vi "Soft_Robot Model_2States.vi"() -> ()   [LabVIEW 2015]
uses:
  <vilib>/addons/Control Design/_Model Construction/Model Typedefs.llb/CD State Space Model (MIMO).ctl
  <vilib>/addons/Control Design/_Model Construction/Model Typedefs.llb/CD General Elements.ctl
  <vilib>/Platform/TimedLoop/XDataNode/timing_clust.ctl
  <vilib>/Platform/TimedLoop/XDataNode/nitl_modes.ctl
  <vilib>/Platform/TimedLoop/XDataNode/wakeup.ctl
  <vilib>/FPGAPlugInAG/myRIO-1900/niLvFpga_Open_myRIO-1900.vi
  <vilib>/rvi/interface/common/dynamic/niFpgaDynamicAddResources.vi
  <vilib>/Utility/error.llb/Error Cluster From Error Code.vi
  <vilib>/rvi/errors/niLvFpgaAdjustHostInterfaceError.vi
  <vilib>/FPGAPlugInAG/Dynamic/niLvFpga_Close_Dynamic.vi
  <vilib>/Analysis/7linalg.llb/Create Special Real Matrix.vi
  <vilib>/addons/Control Design/_Model Construction/Model Creation.llb/Model Creation SubVI/cd_Create State Space Model.vi
  <vilib>/addons/Control Design/_State Feedback Control/State Feedback Control.llb/State Feedback Control SubVis/cd_Linear Quadratic Regulator.vi
  <vilib>/addons/Control Design/_Stochastic Systems/Stochastic Systems.llb/CD Construct Noise Model (Numeric).vi
  <vilib>/Simulation/Estimation/Implementation/NILVSim Discrete Kalman Filter.llb/SIM Disc KF Pred and Corr with Pred Gain with Checking Direct LV.vi
  <vilib>/rvi/interface/nirviOpenFPGA/nirviOpenFPGA.xnode
  FPGA Bitfiles/ACC20115_FPGATarget_CurrentControlle_Dt5vFgOzYtY.lvbitx
  Current Controller.vi
  <vilib>/rvi/interface/nirviReadWriteControl/nirviReadWriteControl.xnode
  <vilib>/rvi/interface/nirviCloseFPGA/nirviCloseFPGA.xnode
  <vilib>/Platform/TimedLoop/XDataNode/XDataNode.xnode
  <vilib>/Simulation/Implementation/XNodeFramework/SimXNode/SimX.xnode
  NiFpgaLv.dll
  <vilib>/rvi/interface/Simulation/niFpgaSimulationCallBeginRW.vi
  <vilib>/addons/Control Design/_State Feedback Control/NI_CD_State Feedback Control.lvlib
  <vilib>/addons/Control Design/_Stochastic Systems/NI_CD_Stochastic Systems.lvlib
  <vilib>/Platform/TimedLoop/XDataNode/XDNodeRunTimeDep.lvlib
  <vilib>/Analysis/NI_AALPro.lvlib
  <vilib>/addons/Control Design/_Model Construction/NI_LinSys_Model Creation.lvlib
  <vilib>/addons/Control Design/_Model Construction/NI_LinSys_Model Typedefs.lvlib
panel:
  in  "Tab Control":enum32{"Outputs/Control", "Model Info"}(tab)
  out "DAC Inlet Valve 2":i32(graph)
  out "Fusion Data":dbl(graph)
  out "KF estimate":dbl[](graph)
  in  "SP1:":dbl(slide)=40.87020302841148 min=0.0 max=0.0 scale=0.0..720.0
  in  "Stop":bool
  out "Status?":bool
  in  "Current (mA)":i32
  out "State-Space Model":T1 {"Transport Delay" format="%.2f"; "D" format="%#.2g"; "C" format="%#.2g"; "B" format="%#.2g"; "A" format="%#.2g"; "properties"."Sampling Time" format="%#.6p"; "properties"."Output Delays" format="%.4f"; "properties"."Input Delays" format="%.4f"}
  in  "LQR State Weight Matrix (Q)":dbl[](array[slide])=[1.133823501217849, 15.19911082952933] scale=0.001..1000.0
  in  "LQR Output weighting matrix (R)":dbl[](array[slide])=[0.061359072734131735] scale=0.0001..10.0
  in  "A":dbl[][](array[numeric]) format="%#.5g"
  in  "B":dbl[][](array[numeric]) format="%#.5g"
  in  "C":dbl[][](array[numeric]) format="%#.5g"
  in  "D":dbl[][](array[numeric]) format="%#.5g"
  in  "KF Q":dbl[][](array[numeric]) format="%#.2g"
  in  "KF R":dbl[][](array[numeric]) format="%#.2g"
  in  "KF P(0|-1)":dbl[][](array[numeric])=[[1.0]]
  in  "Stoch. K":dbl[][](array[numeric]) format="%#.2g"
  out "error IO":errorcluster
  in  "xhat(0|-1)":dbl[](array[numeric])=[1.0]
  out "error out":errorcluster
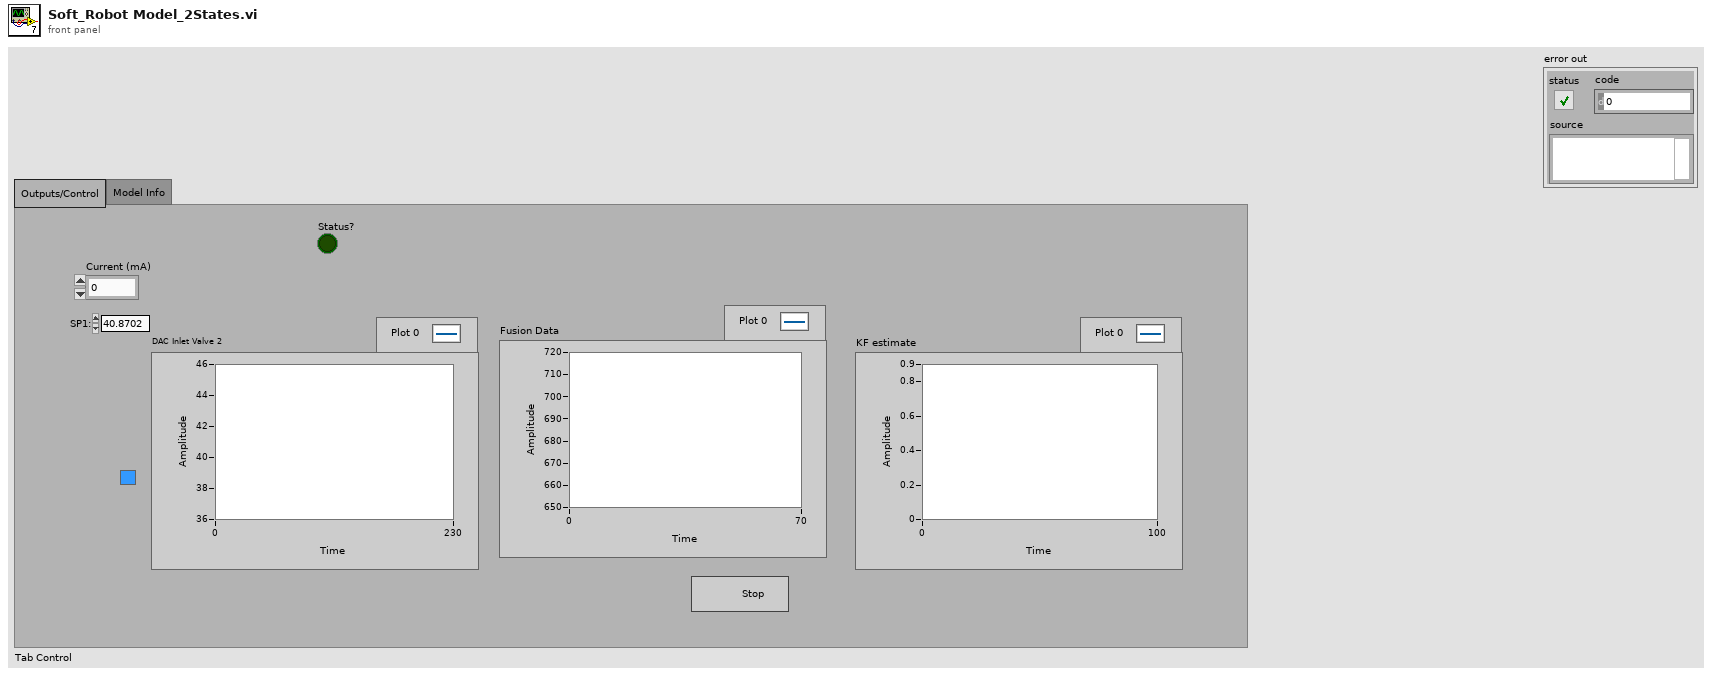
[diagram p1: front panel]
types:
  T1 = typedef "NI_LinSys_Model Typedefs.lvlib/CD State Space Model (MIMO).ctl" = cluster{"properties":T2, "A":dbl[][], "B":dbl[][], "C":dbl[][], "D":dbl[][], "StateNames":string[], "Transport Delay":dbl[][]}
  T2 = typedef "NI_LinSys_Model Typedefs.lvlib/CD General Elements.ctl" = cluster{"Model name":string, "Input names":string[], "Output names":string[], "Input Delays":dbl[], "Output Delays":dbl[], "Sampling Time":dbl, "Notes":string}
  T3 = typedef "XDNodeRunTimeDep.lvlib/timing_clust.ctl" = cluster{"Expected End [f-1]":u64, "Actual End [f-1]":u64, "Finished Late? [f-1]":bool, "Expected End [i-1]":u64, "Actual End [i-1]":u64, "Finished Late? [i-1]":bool, "Expected Start [i]":u64, "Actual Start [i]":u64, "Expected Start [f]":u64, "Actual Start [f]":u64, "Source Name":string, "Structure Name":string, "Period":i64, "Deadline":i64, "Offset":i64, "Start":i64, "Priority":i32, "Timeout":i32, "Mode":T4, "Wakeup Reason":T5, "Error":errorcluster, "Source Type":string, "Secondary Source Type":string, "Global End Time":u64, "Global Start Time":u64, "Frame Duration":u64, "Iteration Duration":u64, "Assigned CPU":i32, "I/O Scan Engine Mode":u32}
  T4 = typedef "XDNodeRunTimeDep.lvlib/nitl_modes.ctl" = enum32{"No Change", "Process missed periods, maintain original phase", "Discard missed periods, maintain original phase", "Process missed periods, ignore original phase", "Discard missed periods, ignore original phase"}
  T5 = typedef "XDNodeRunTimeDep.lvlib/wakeup.ctl" = enum32{"Normal", "Aborted", "Asynchronous wakeup", "Timing source error", "Timed loop error", "Timeout"}
  T6 = enum16{"state weighting", "output weighting, Dim Q = Ny", "output weighting, Dim Q = Nx"}
  T7 = enum32{"Identity", "Diagonal", "Toepliz", "Vandermonde", "Companion"}
  T8 = typedef "NI_Matrix.lvlib/RealMatrix.ctl" = dbl[][]
  T9 = typedef "NI_CD_Stochastic Systems.lvlib/cd_Stochastic State-Space Model.ctl" = cluster{"Sampling Time (s)":dbl, "G":dbl[][], "B":dbl[][], "A":dbl[][], "C":dbl[][], "D":dbl[][], "H":dbl[][]}
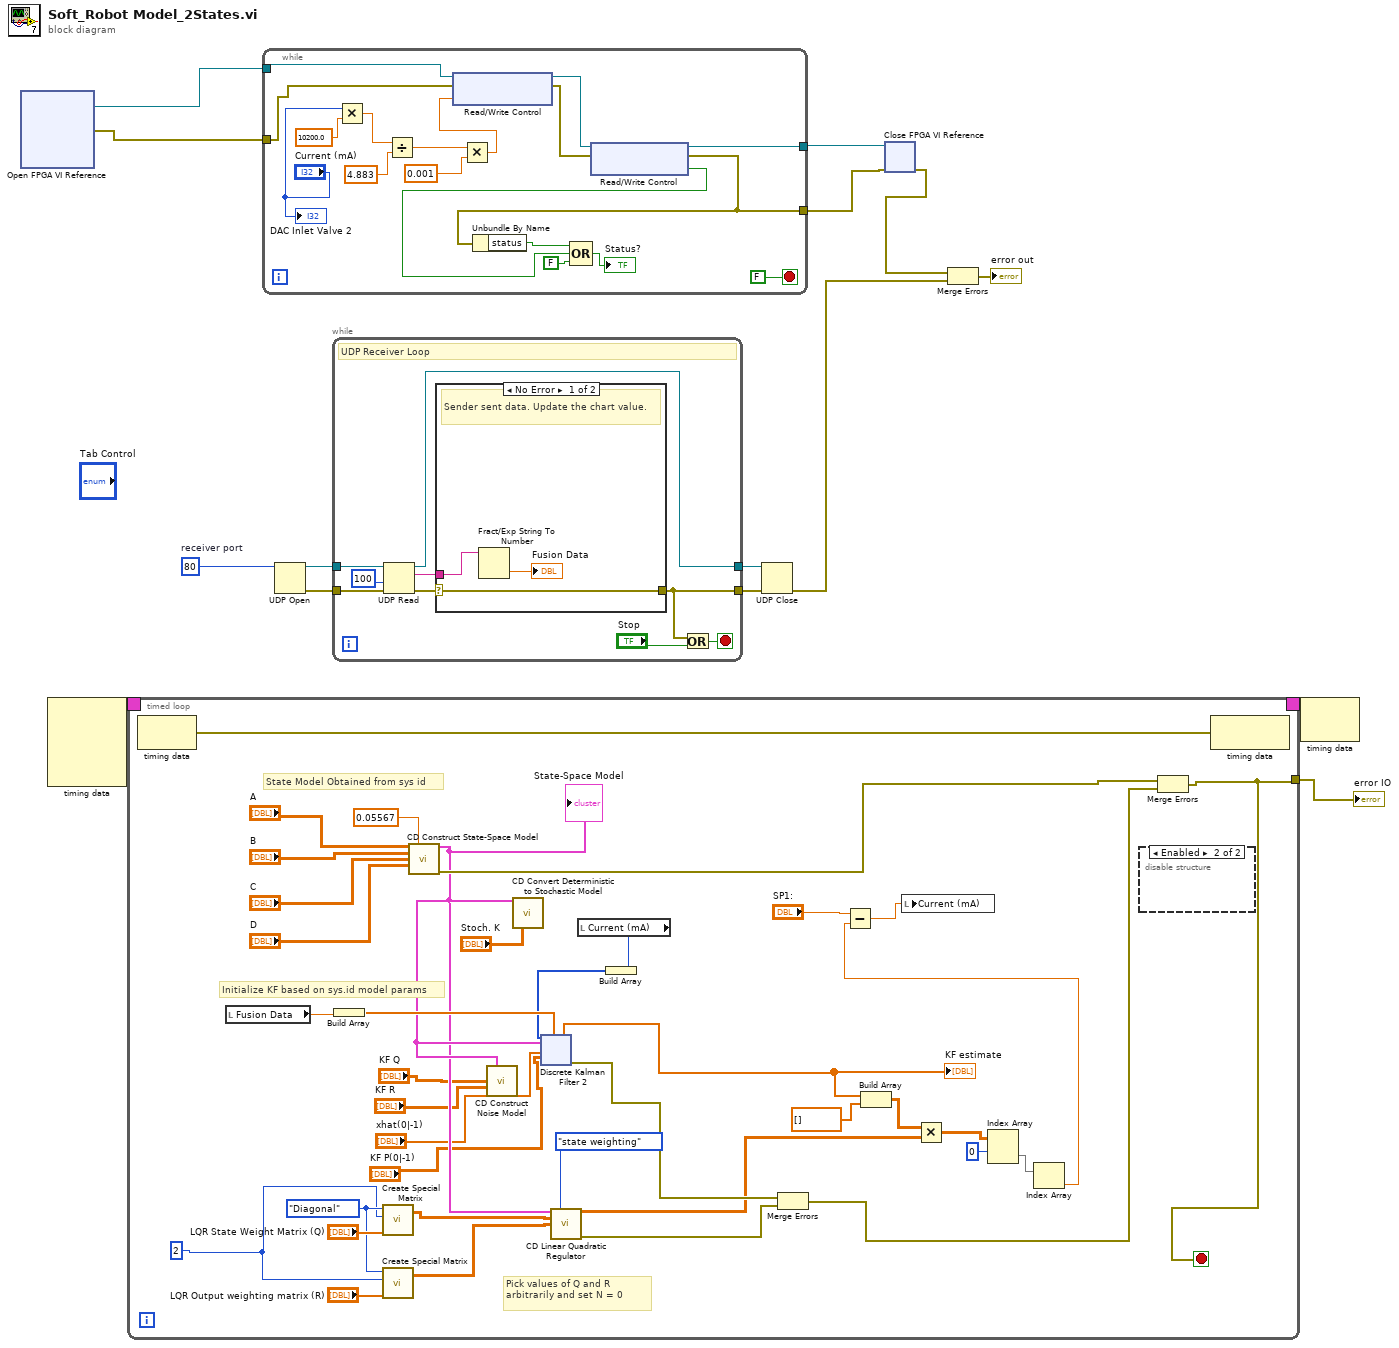
[diagram p0: block diagram]
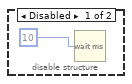
[diagram p2: hidden frame]
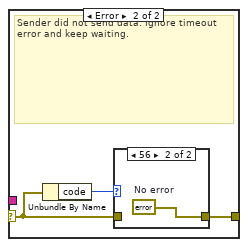
[diagram p3: hidden frame]
diagram:
  w11 = u16 80  # receiver port
  n1 = xnode "Open FPGA VI Reference"() -> ("FPGA VI Reference Out"=w3:refnum<k20>, "error out"=w4:errorcluster)  [unwired: 2 in]
  n2 = node-c288() -> (w2:T3)  [unwired: 4 in]
  n3 = timed-loop {
    tunnel: [w26] -> w5
    timing: w2 -> [_]
    timing-out: [_] -> w1
    stop <- w26 stop-if-true
    w27 = 2
    w34 = T7."Diagonal" ("matrix type")
    # "Pick values of Q and R\narbitrarily and set N = 0"
    # "State Model Obtained from sys id"
    # "Initialize KF based on sys.id model params"
    n4 = node-c288() -> (w25:errorcluster)  [unwired: 1 in]
    n5 = local read "Fusion Data"() -> (w45:dbl)
    n6 = Build Array ("Build Array 6")(w45) -> (w41:dbl[])
    n7 = call-poly <vilib>:"Create Special Matrix.vi"("matrix type"=w34, "matrix size"=w27, "Input Vector1"="LQR State Weight Matrix (Q)") -> ("Special Matrix"=w31:T8)  [unwired: 2 in, 1 out]
    n8 = call-poly <vilib>:"Create Special Matrix.vi"("matrix type"=w34, "matrix size"=w27, "Input Vector1"="LQR Output weighting matrix (R)") -> ("Special Matrix"=w30:T8)  [unwired: 2 in, 1 out]
    n9 = call-poly <vilib>:"CD Construct State-Space Model.vi"("A"="A", "Sampling Time (s)"=0.05567, "B"="B", "C"="C", "D"="D") -> ("State-Space Model"=w32:T1, "error out"=w42:errorcluster)  [unwired: 9 in]
    "State-Space Model" <- w32
    n10 = call <vilib>:"CD Convert Deterministic to Stochastic Model.vi"("Deterministic State-Space Model"=w32, "G"="Stoch. K") -> ("Stochastic State-Space Model"=w38:T9)  [unwired: 12 in, 1 out]
    n11 = call-poly <vilib>:"CD Construct Noise Model.vi"("Stochastic State-Space Model"=w38, "Q"="KF Q", "R"="KF R") -> ()  [unwired: 11 in, 2 out]
    n12 = call-poly <vilib>:"CD Linear Quadratic Regulator.vi"("State-Space Model"=w32, "Weighting Type"=T6."state weighting", "Q"=w31, "R"=w30) -> ("Optimal Gain (K)"=w29:dbl[][], "error out"=w28:errorcluster)  [unwired: 8 in, 2 out]
    n13 = local read "Current (mA)"() -> (w43:i32)
    n14 = Build Array ("Build Array 5")(w43) -> (w37:i32[])
    n15 = xnode ("Discrete Kalman Filter 2")("input u(k)"=w37, "Stochastic State-Space Model"=w38, "Initial State Estimate xhat(0|-1)"="xhat(0|-1)", "Initial Estimation Error Covariance P(0|-1)"="KF P(0|-1)", "Output y(k)"=w41) -> ("Estimated Output yhat(k)"=w40:dbl[], "error out"=w39:errorcluster)  [unwired: 3 in, 6 out]
    "KF estimate" <- w40
    n16 = Merge Errors(w39, w28) -> (w48:errorcluster)
    n17 = Build Array ("Build Array 9")(w40, dbl[] [] ("element")) -> (w50:dbl[][])
    n18 = Multiply(x=w50, y=w29) -> (x*y=w52:dbl[][])
    n19 = Index Array(array=w52, index (row)=0) -> (element=w54:dbl[])  [unwired: 1 in]
    n20 = Index Array ("Index Array 2")(array=w54) -> (element=w46:dbl)  [unwired: 1 in]
    n21 = Subtract(x="SP1:", y=w46) -> (x-y=w44:dbl)
    n22 = local write "Current (mA)"(w44) -> ()
    n23 = disable-structure shown="Enabled" {
      frame Disabled {
        n24 = Wait (ms)(milliseconds to wait=u32 10 ("millisecond timer value")) -> ()  [unwired: 1 out]
      }
      frame Enabled {
      }
    }
    n25 = Merge Errors(w42, w48) -> (w26:errorcluster)
    n26 = node-c288(w25) -> ()  [unwired: 1 out]
  }
  "error IO" <- w5
  n27 = while {
    tunnel: w3 -> [w93]
    tunnel: w4 -> [w77]
    tunnel: [w87] -> w9
    tunnel: [w85] -> w10
    stop <- FALSE stop-if-true
    n28 = Multiply(x="Current (mA)", y=10200.0) -> (x*y=w80:dbl)
    n29 = Divide(x=w80, y=4.883) -> (x/y=w83:dbl)
    n30 = Multiply(x=w83, y=0.001) -> (x*y=w79:dbl)
    n31 = xnode "Read/Write Control"("FPGA VI Reference In"=w93, "error in"=w77, "DAC Inlet Valve"=w79) -> ("FPGA VI Reference Out"=w92:refnum<k20>, "error out"=w91:errorcluster)
    n32 = xnode "Read/Write Control"("FPGA VI Reference In"=w92, "error in"=w91) -> ("FPGA VI Reference Out"=w85:refnum<k20>, "error out"=w87:errorcluster, "Inlet Overflow?"=w86:bool)
    n33 = Unbundle By Name(w87) -> ("status"=w89:bool)
    n34 = Compound Arithmetic op=OR(w89, w86, FALSE ("value")) -> (→"Status?":bool)
    "DAC Inlet Valve 2" <- "Current (mA)"
  }
  n35 = UDP Open(11:w11) -> (port=w12:refnum<k16>, 0:w13:errorcluster)  [unwired: 4 in, 1 out]
  n36 = while {
    tunnel: w12 -> [w103]
    tunnel: [w95] -> w15
    tunnel: w13 -> [w100]
    tunnel: [w96] -> w14
    stop <- w101 stop-if-true
    # "UDP Receiver Loop"
    n37 = UDP Read(connection ID=w103, timeout ms (25000)=100, 8:w100) -> (data out=w98:string, error out=w97:errorcluster, 3:w95:refnum<k16>)  [unwired: 3 out]
    n38 = case shown="No Error" w97 {
      selector: w97 -> [w104 w108]
      tunnel: w98 -> [w106 _]
      tunnel: [w104 w107] -> w96
      frame No Error {
        # "Sender sent data. Update the chart value."
        n39 = Fract/Exp String To Number(string=w106) -> (number=→"Fusion Data":dbl)  [unwired: 3 in, 1 out]
      }
      frame Error {
        # "Sender did not send data. Ignore timeout error and keep waiting."
        n40 = Unbundle By Name(w108) -> ("code"=w109:i32)
        n41 = case shown="56" w109 {
          tunnel: w108 -> [w110 _]
          tunnel: [w110 w111] -> w107
          frame Default {
          }
          frame 56 {
            w111 = errorcluster {"status"=FALSE, "code"=0, "source"=""}  # No error
          }
        }
      }
    }
    n42 = Or(x=w96, y="Stop") -> (x .or. y?=w101:bool)
  }
  n43 = UDP Close(connection ID=w15, 8:w14) -> (error out=w7:errorcluster)  [unwired: 1 out]
  n44 = xnode "Close FPGA VI Reference"("FPGA VI Reference In"=w10, "error in"=w9) -> ("error out"=w8:errorcluster)
  n45 = Merge Errors(w8, w7) -> (→"error out":errorcluster)
  n46 = node-c288(w1) -> ()  [unwired: 1 out]
